vi "EventStopOnTrack.vi"(6 "Track ID":u64, 8 "error in":errorcluster) -> (0 "error out":errorcluster)   [LabVIEW 2024, in "VS_Perfetto.lvlib"]
uses:
  VS_Perfetto.lvlib
  libvs_perfetto.dll
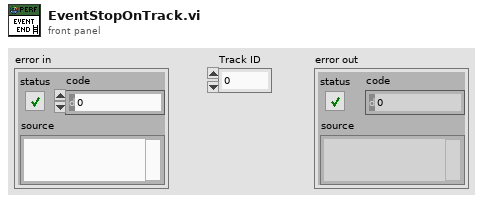
[diagram p1: front panel]
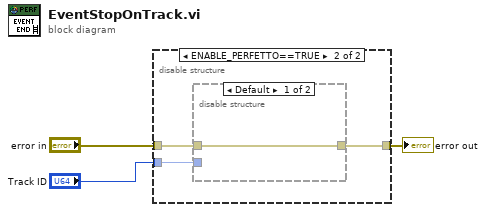
[diagram p0: block diagram]
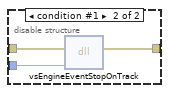
[diagram p3: hidden frame]
diagram:
  n1 = disable-structure shown="ENABLE_PERFETTO==TRUE" {
    disable-tunnel: "error in" -> [w4 w6]
    disable-tunnel: [w4 w7] -> w2
    disable-tunnel: "Track ID" -> [_ w5]
    frame condition #0 (active) {
    }
    frame condition #1 {
      n2 = disable-structure shown="Default" {
        disable-tunnel: [w8 w10] -> w7
        disable-tunnel: w6 -> [w8 w11]
        disable-tunnel: w5 -> [_ w9]
        frame condition #0 (active) {
        }
        frame condition #1 {
          n3 = dll-call lib="libvs_perfetto.*" fn="vsEngineEventStopOnTrack"(error in=w11, "trackId"=w9) -> (error out=w10:errorcluster)  [unwired: 4 in, 1 out]
        }
      }
    }
  }
  "error out" <- w2
